vi "I2C Controller Module.vi"(11 "error in (no error)":errorcluster) -> (15 "error out":errorcluster)   [LabVIEW 2020, in "I2C Controller Lib.lvlib"]
uses:
  I2C Controller Lib.lvlib
  TypeDef/Transmission Data.ctl
  TypeDef/DVR Cluster.ctl
  Class/Transmission Mode/Parent/TX Speed.lvclass
  Class/Addressing Mode/Parent/Addressing Mode.lvclass
  Class/Devices/Parent/Devices.lvclass
  TypeDef/Path Cluster.ctl
  TypeDef/Queue Operation Mode.ctl
  TypeDef/User LV2 Mode Select.ctl
  <vilib>/Utility/config.llb/Read Key (String).vi
  Class/Transmission Mode/Child/Low Speed/SubVI/SubPanel.vi
  <vilib>/Utility/config.llb/NI_LVConfig.lvlib
  Class/Transmission Mode/Child/Low Speed/Low Speed.lvclass
panel:
  in  "Clear?":bool
  in  "Configure?":bool
  out "Warning":string caption="Warning:"
  in  "TX.Data":T1=[10, 188, 218, 14, 47, 69, 255, 107, 7, 92, 64] caption="Transmission Data" format="%.0x"
  out "RX.Data":u8[](array[numeric]) caption="Read Bytes" format="%.0x"
  out "Acknoledge?":bool caption="ACK / NACK"
  in  "Speed Mode":string(combo)="Select Device"
  in  "Transmit Data?":bool caption="Start Transmission"
  in  "Add Device?":bool caption="Add DEvice?"
  in  "Oper. Mode":string(combo)="Select Operation" caption="Operation Mode"
  in  "Address Mode":enum32{"7-bit", "10-Bit"}(radio) caption="Addressing Mode"
  in  "Log.Open?":bool
  in  "Target Address":u16 max=128 step=1 format="%.0x"
  in  "Device Type":string(combo)="Select Device Type"
  in  "Voltage":dbl=1.8 caption="Voltage (V)" min=1.8 max=5.0 step=1.0 format="%.2g"
  out "Digital Waveform Graph":digitaldata[](graph) caption="Graph"
  # "I2C Controller Module"
  # "Controller"
  # "Target"
  # "Transmission Parameters"
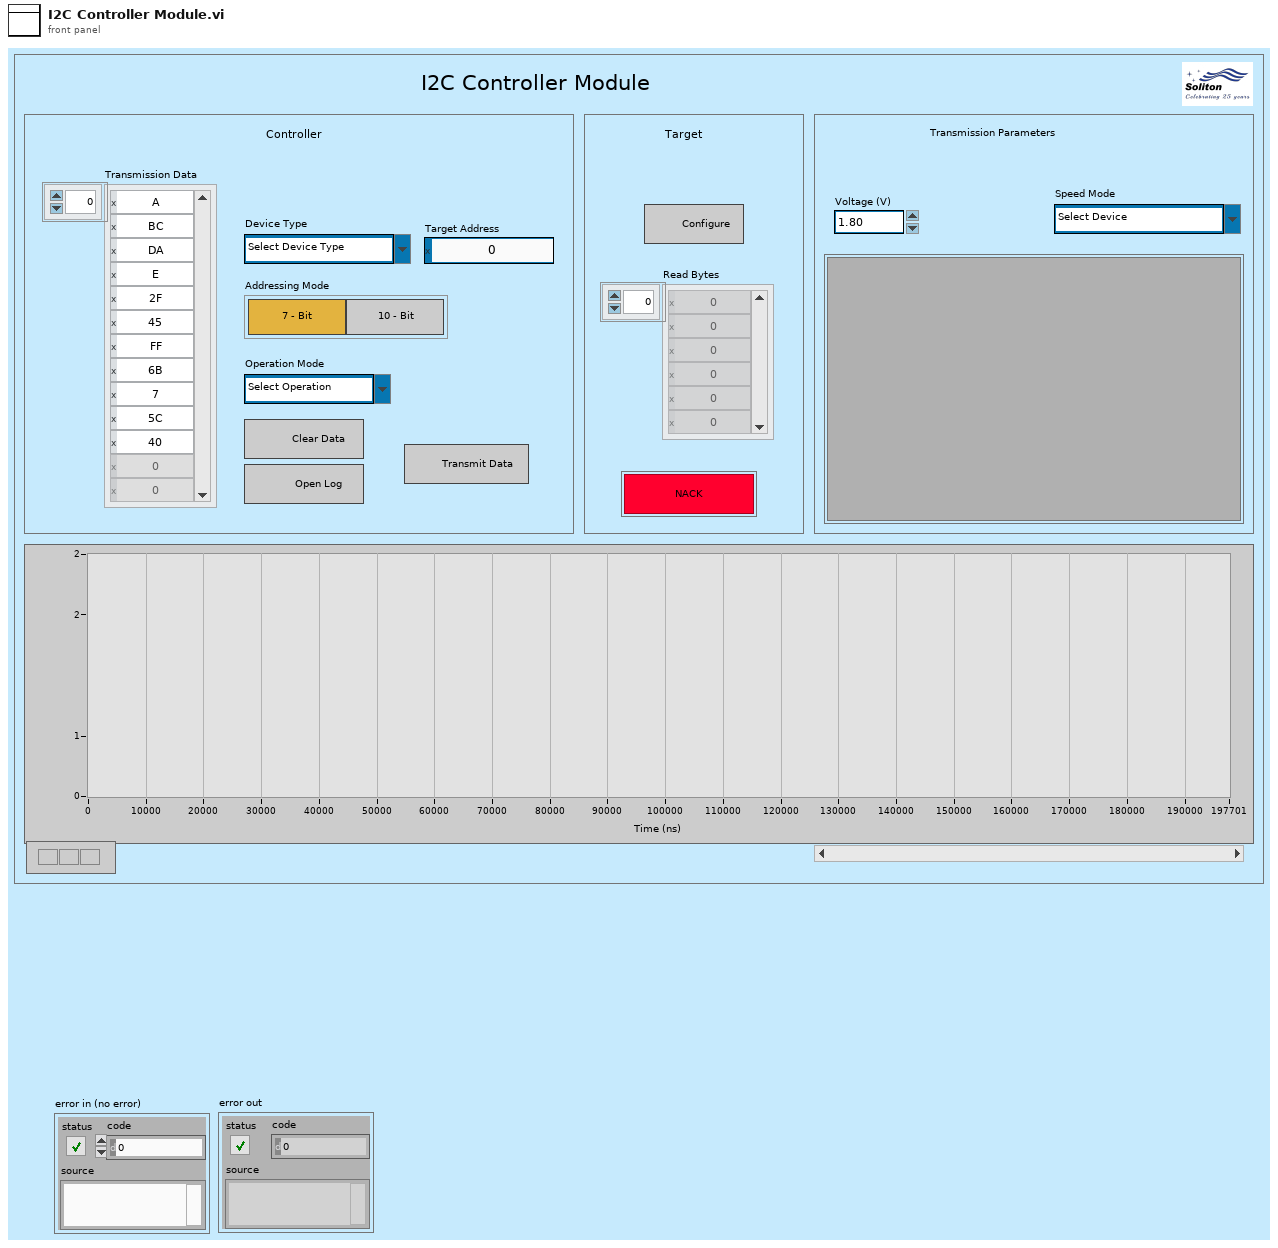
[diagram p1: front panel]
types:
  T1 = typedef "I2C Controller Lib.lvlib/Transmission Data.ctl" = u8[]
  T2 = typedef "I2C Controller Lib.lvlib/User LV2 Mode Select.ctl" = enum16{"Create", "Delete", "Stop"}
  T3 = typedef "I2C Controller Lib.lvlib/Queue Operation Mode.ctl" = enum16{"Create Q", "Enqueue", "Enqueue N", "Enstack", "Dequeue", "Flush Q", "Close Q"}
  T4 = typedef "I2C Controller Lib.lvlib/DVR Cluster.ctl" = cluster{"TX. Mode":refnum<data-value>, "Addr. Mode":refnum<data-value>, "Devices":refnum<data-value>}
  T5 = typedef "I2C Controller Lib.lvlib/Path Cluster.ctl" = cluster{"Config File":path, "TX.Mode":path, "Devices":path, "Addr. Mode":path}
  T6 = cluster{"Enable/Disable":string, "Warning":string, "Oper. Mode":string, "Speed Mode":string, "Address Mode":enum32{"7-bit", "10-Bit"}, "TX.Data":T1, "Device Type":string, "DVR":T4, "Path":T5, "Flags":cluster{"Device Type":bool, "Speed Mode":bool, "Target Address":bool, "Oper. Mode":bool}, "RX.Data":u8[], "Acknoledge?":bool, "Graph Wave":digitaldata[]}
  T7 = typedef "NI_LVConfig.lvlib/Config Data RefNum.ctl" = refnum<k1>
  T8 = enum8{"Enabled", "Disabled", "Disabled and Grayed Out"}
  T9 = cluster{"Device Type":bool, "Speed Mode":bool, "Target Address":bool, "Oper. Mode":bool}
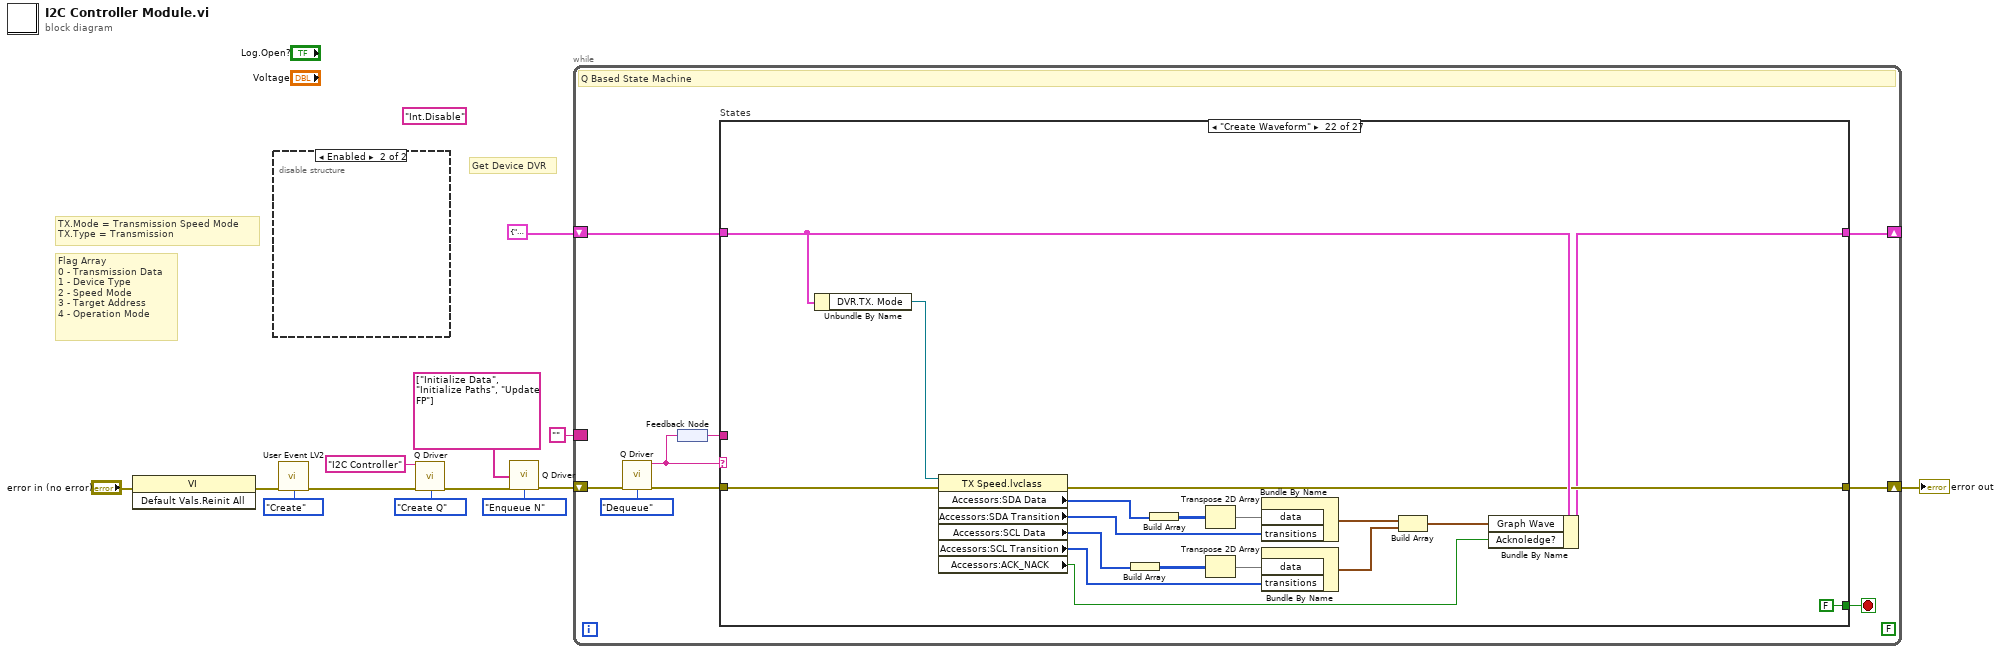
[diagram p0: block diagram]
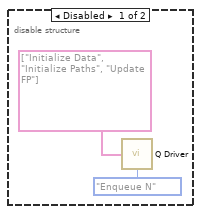
[diagram p2: hidden frame]
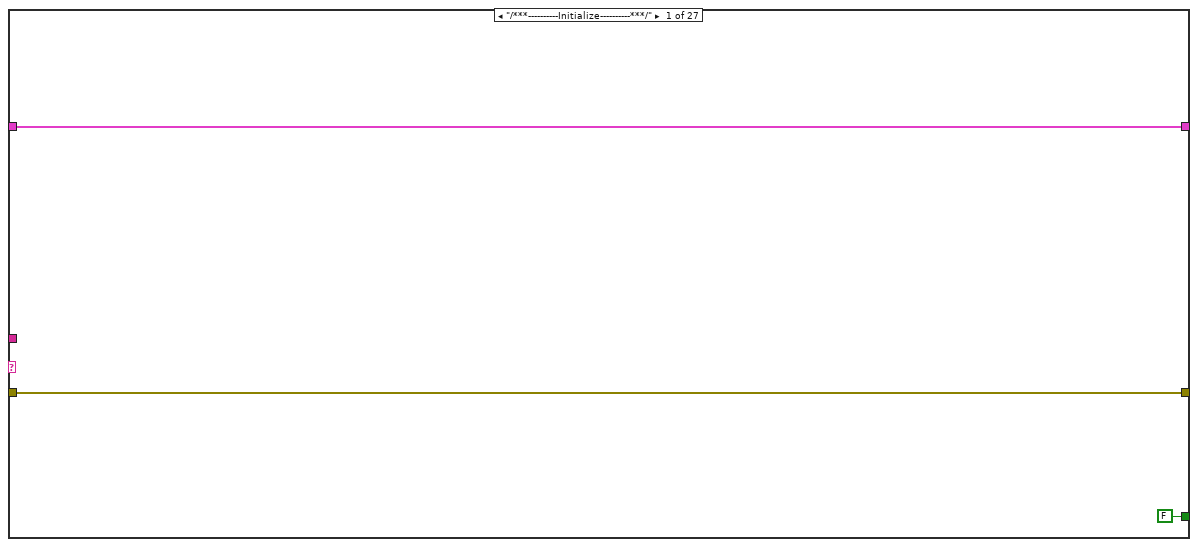
[diagram p3: hidden frame]
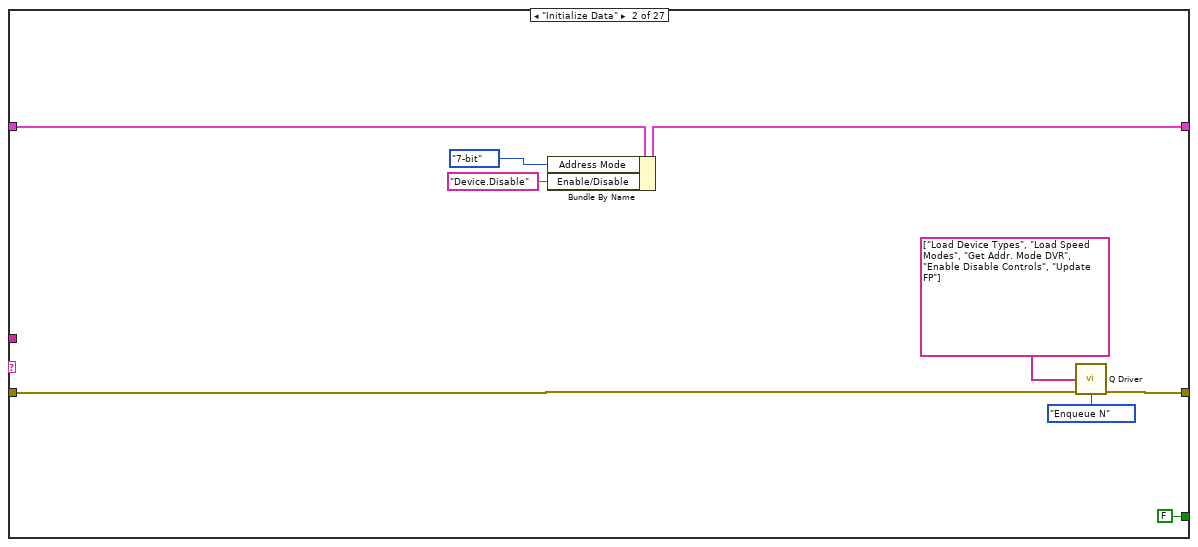
[diagram p4: hidden frame]
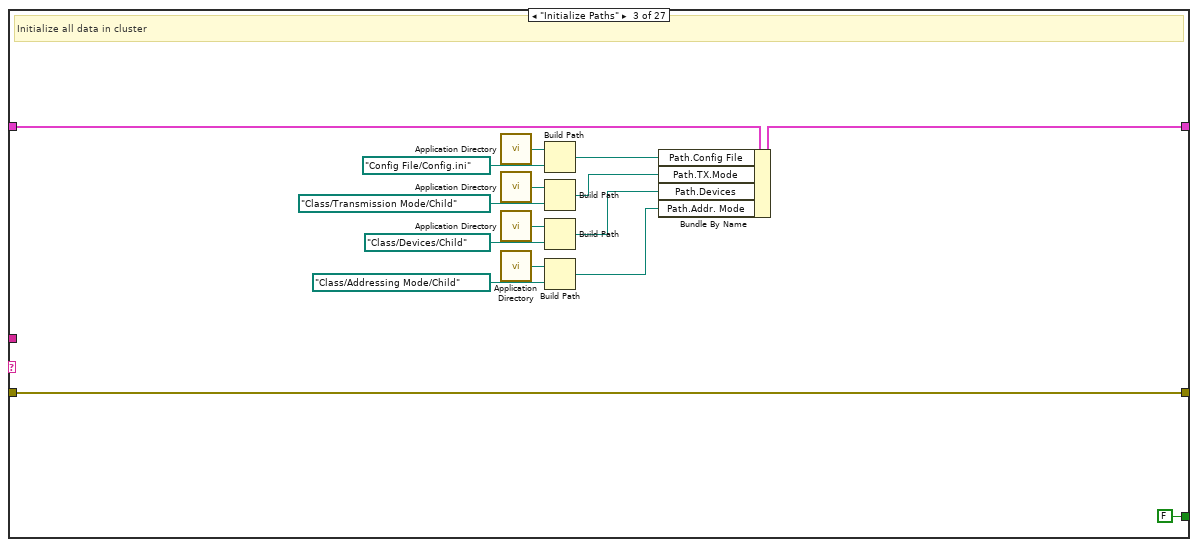
[diagram p5: hidden frame]
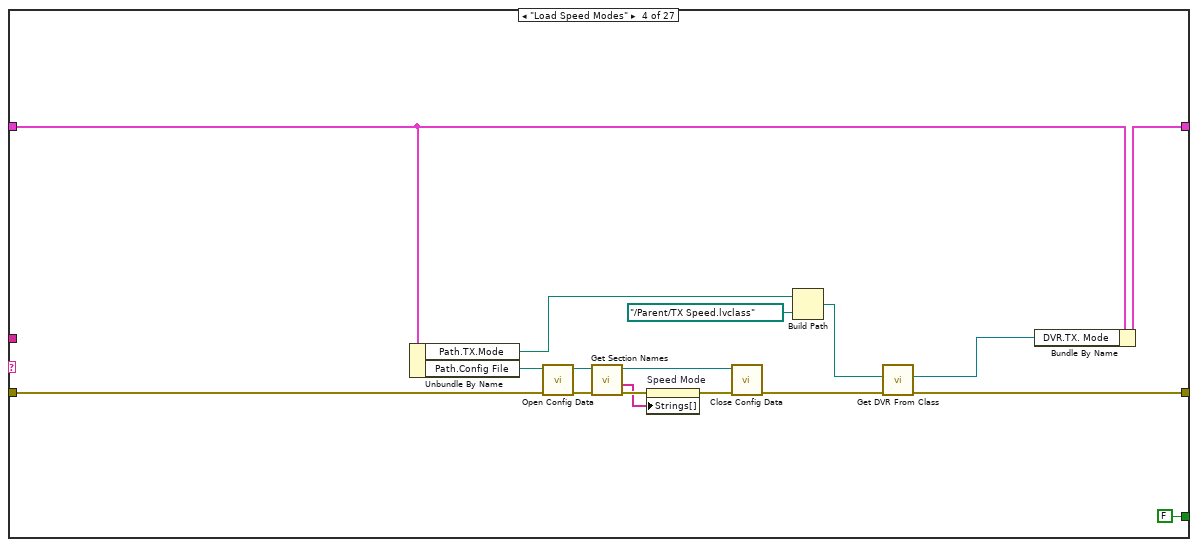
[diagram p6: hidden frame]
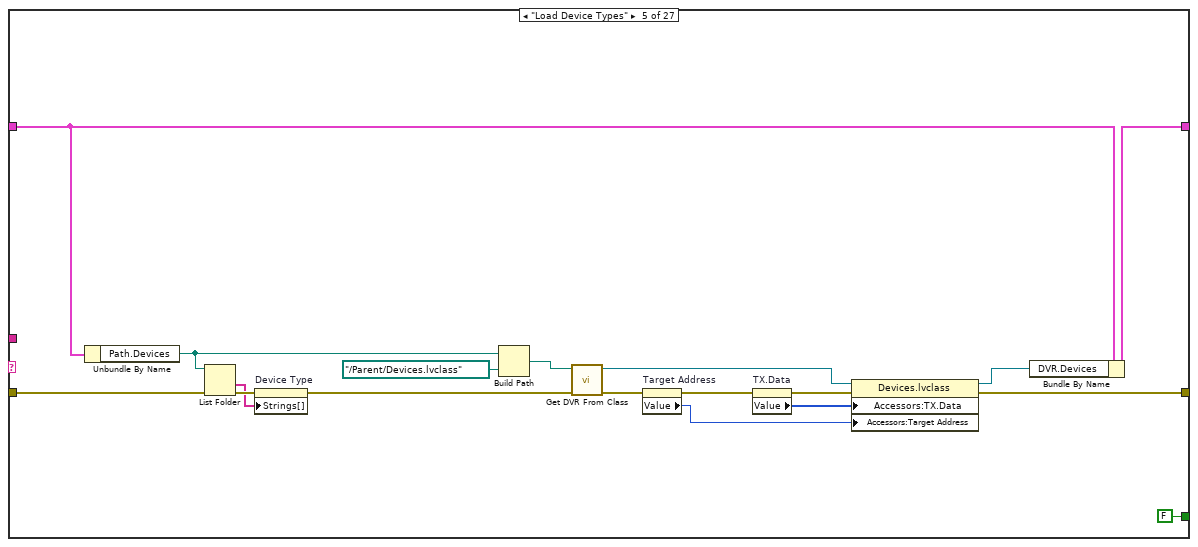
[diagram p7: hidden frame]
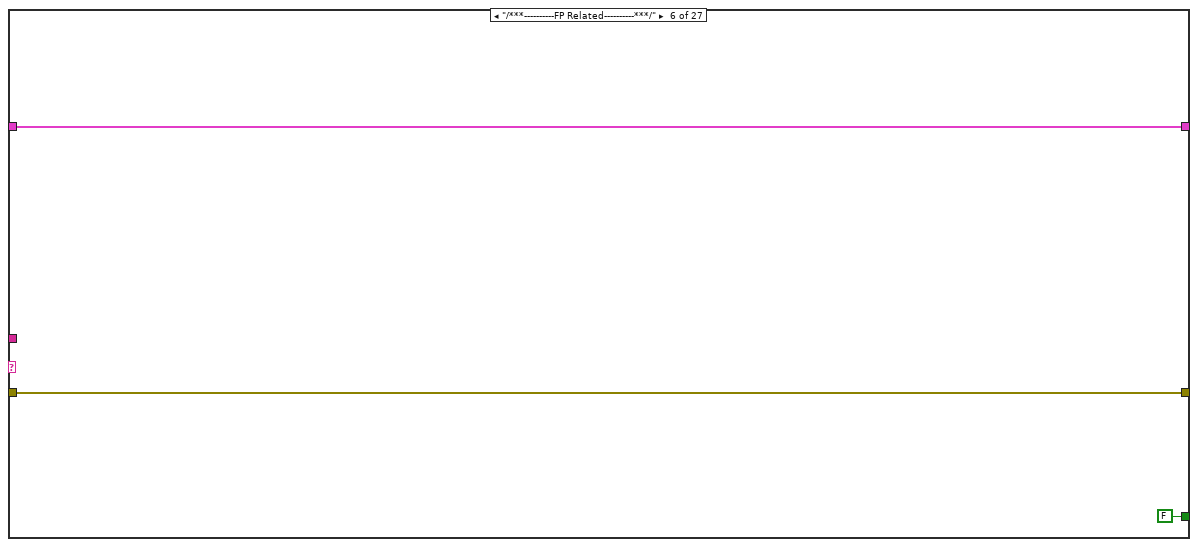
[diagram p8: hidden frame]
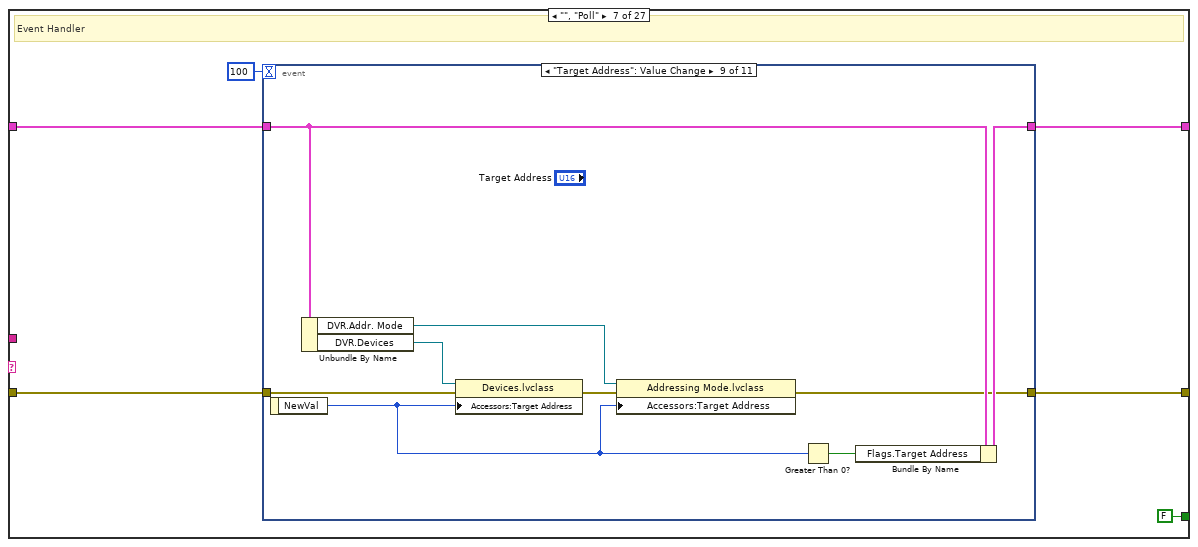
[diagram p9: hidden frame]
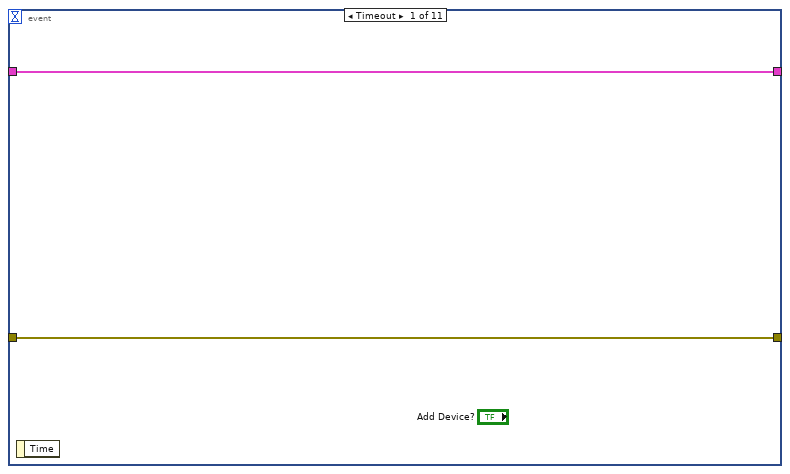
[diagram p10: hidden frame]
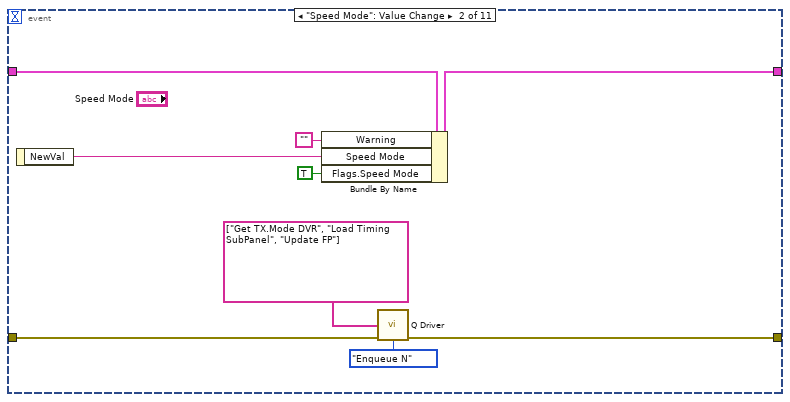
[diagram p11: hidden frame]
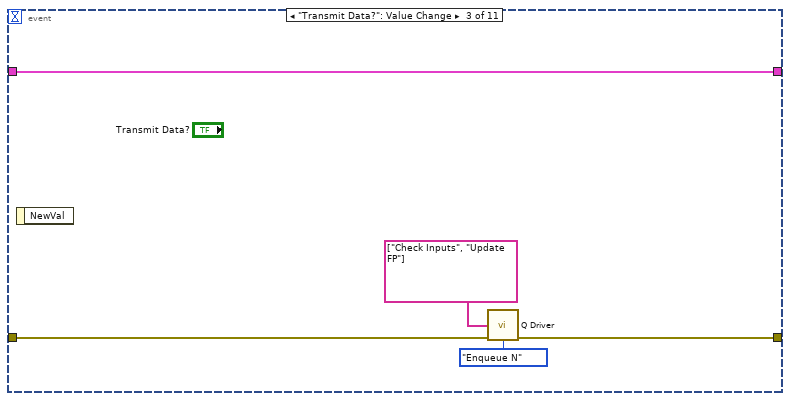
[diagram p12: hidden frame]
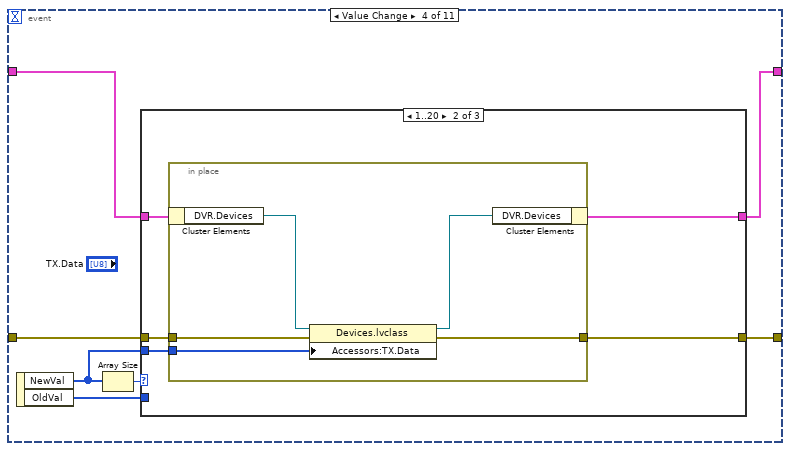
[diagram p13: hidden frame]
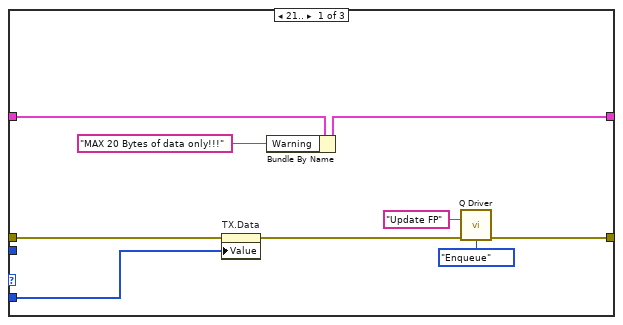
[diagram p14: hidden frame]
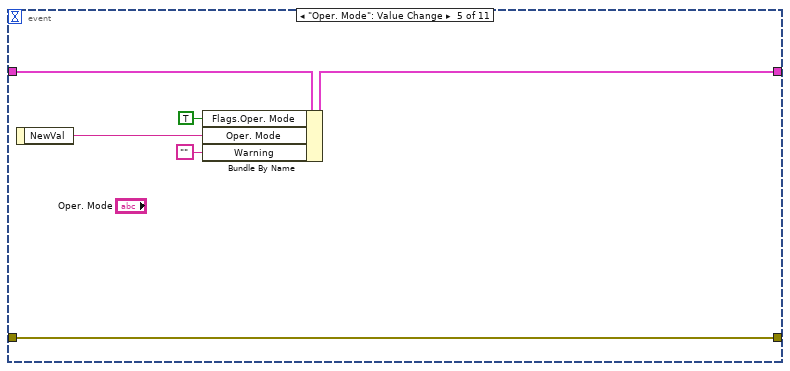
[diagram p16: hidden frame]
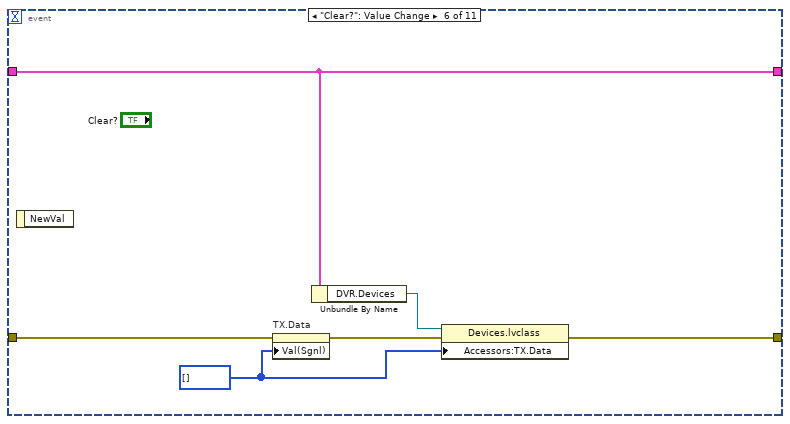
[diagram p17: hidden frame]
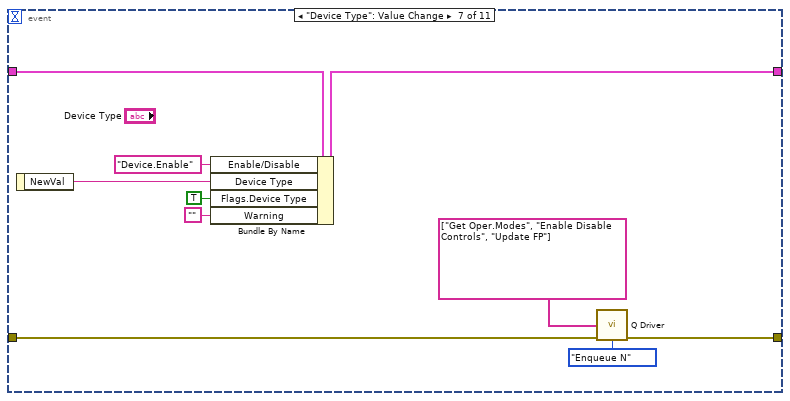
[diagram p18: hidden frame]
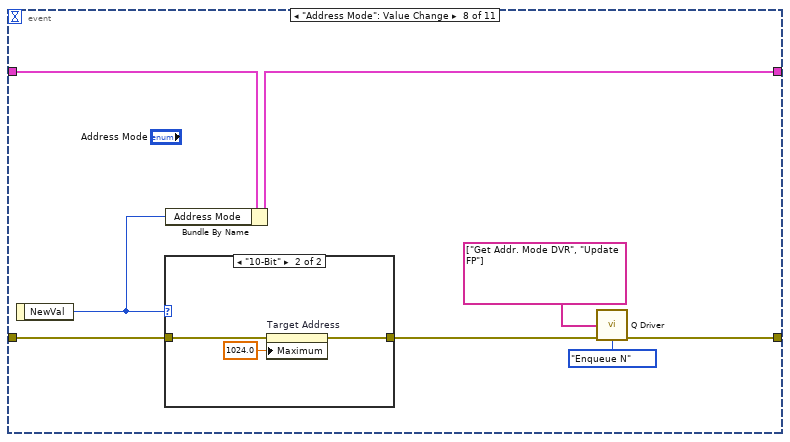
[diagram p19: hidden frame]
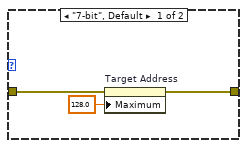
[diagram p20: hidden frame]
diagram:
  (unwired) "Int.Disable" ("Enable/Disable")
  # "Get Device DVR"
  # "Flag Array\n0 - Transmission Data\n1 - Device Type\n2 - Speed Mode\n3 - Target Address\n4 - Operation Mode"
  # "TX.Mode = Transmission Speed Mode\nTX.Type = Transmission"
  n1 = invoke class="VI" method="Default Vals.Reinit All"(error in="error in (no error)") -> (error out=w2:errorcluster)  [unwired: 2 in, 2 out]
  n2 = disable-structure shown="Enabled" {
    frame Disabled {
      n3 = call "Q Driver.vi"("States s[]"=string[] ["Initialize Data", "Initialize Paths", "Update FP"], "Q Operation"=Queue_Operation_Mode."Enqueue N") -> ()  [unwired: 12 in, 2 out]
    }
    frame Enabled {
    }
  }
  n4 = call "User Event LV2.vi"("error in (no error)"=w2, "LV2 Mode"=User_LV2_Mode_Select."Create") -> ("error out"=w1:errorcluster)  [unwired: 12 in, 1 out]
  n5 = call "Q Driver.vi"("Q Name"="I2C Controller", "error in (no error)"=w1, "Q Operation"=Queue_Operation_Mode."Create Q") -> ("error out"=w12:errorcluster)  [unwired: 11 in, 1 out]
  n6 = call "Q Driver.vi"("States s[]"=string[] ["Initialize Data", "Initialize Paths", "Update FP"], "error in (no error)"=w12, "Q Operation"=Queue_Operation_Mode."Enqueue N") -> ("error out"=w11:errorcluster)  [unwired: 11 in, 1 out]
  n7 = while {
    shift-right: [w21] -> _
    shift-left: T6 {"Enable/Disable"="", "Warning"="", "Oper. Mode"="", "Speed Mode"="", "Address Mode"=enum."7-bit", "TX.Data"=[], "Device Type"="", "DVR"={"TX. Mode"=refnum, "Addr. Mode"=refnum, "Devices"=refnum}, "Path"={"Config File"=path "", "TX.Mode"=path "", "Devices"=path "", "Addr. Mode"=path ""}, "Flags"={"Device Type"=FALSE, "Speed Mode"=FALSE, "Target Address"=FALSE, "Oper. Mode"=FALSE}, "RX.Data"=[], "Acknoledge?"=FALSE, "Graph Wave"=[]} -> [w20]
    shift-right: [w22] -> w8
    shift-left: w11 -> [w24]
    border: "" -> [_]
    stop <- w19 stop-if-true
    (unwired) FALSE
    (unwired) FALSE
    # "Q Based State Machine"
    n8 = call "Q Driver.vi"("error in (no error)"=w24, "Q Operation"=Queue_Operation_Mode."Dequeue") -> ("State Out"=w17:string, "error out"=w23:errorcluster)  [unwired: 12 in]
    n9 = feedback-in #1(w17) -> ()
    n10 = feedback #1() -> (w16:string)
    n11 = case "States" shown="\"Create Waveform\"" w17 {
      selector: w17 -> [_ _ _ _ _ _ _ _ _ _ _ _ _ _ _ _ _ _ _ _ _ _ _ _ w490 _ _]
      tunnel: w23 -> [w27 w31 w40 w68 w86 w90 w96 w213 w233 w236 w242 w272 w288 w308 w319 w325 w332 w351 w366 w394 w447 w465 w468 w471 w492 w513 w518]
      tunnel: [w27 w30 w40 w55 w75 w90 w95 w214 w233 w236 w244 w274 w285 w308 w318 w324 w331 w351 w358 w392 w436 w463 w468 w470 w491 w513 w516] -> w22
      tunnel: [w26 w35 w50 w54 w80 w89 w93 w212 w231 w235 w243 w275 w290 w307 w320 w323 w330 w350 w361 w395 w434 w451 w467 w482 w503 w512 w520] -> w21
      tunnel: w20 -> [w26 w36 w51 w61 w85 w89 w92 w212 w231 w235 w250 w273 w287 w307 w320 w323 w330 w350 w361 w397 w444 w464 w467 w482 w503 w512 w520]
      tunnel: [FALSE FALSE FALSE FALSE FALSE FALSE FALSE FALSE FALSE FALSE FALSE FALSE FALSE FALSE FALSE FALSE FALSE FALSE FALSE FALSE FALSE FALSE FALSE FALSE FALSE FALSE TRUE] -> w19
      tunnel: w16 -> [_ _ _ _ _ _ _ _ _ _ _ _ _ _ _ _ _ _ _ _ _ _ _ w469 _ _ _]
      frame "/***----------Initialize----------***/" {
      }
      frame "Initialize Data" {
        n12 = Bundle By Name(cluster=w36, "Address Mode"=enum32{"7-bit", "10-Bit"}."7-bit", "Enable/Disable"="Device.Disable") -> (w35:T6)
        n13 = call "Q Driver.vi"("States s[]"=string[] ["Load Device Types", "Load Speed Modes", "Get Addr. Mode DVR", "Enable Disable Controls", "Update FP"], "error in (no error)"=w31, "Q Operation"=Queue_Operation_Mode."Enqueue N") -> ("error out"=w30:errorcluster)  [unwired: 11 in, 1 out]
      }
      frame "Initialize Paths" {
        # "Initialize all data in cluster"
        n14 = call <vilib>:"Application Directory.vi"() -> ("Application Directory"=w49:path)
        n15 = call <vilib>:"Application Directory.vi"() -> ("Application Directory"=w45:path)
        n16 = call <vilib>:"Application Directory.vi"() -> ("Application Directory"=w43:path)
        n17 = call <vilib>:"Application Directory.vi"() -> ("Application Directory"=w39:path)
        n18 = Build Path(base path=w49, name or relative path=path "Config File/Config.ini" ("Config.ini")) -> (appended path=w47:path)
        n19 = Build Path(base path=w45, name or relative path=path "Class/Transmission Mode/Child" ("Config.ini")) -> (appended path=w44:path)
        n20 = Build Path(base path=w43, name or relative path=path "Class/Devices/Child" ("Config.ini")) -> (appended path=w41:path)
        n21 = Build Path(base path=w39, name or relative path=path "Class/Addressing Mode/Child" ("Config.ini")) -> (appended path=w37:path)
        n22 = Bundle By Name(cluster=w51, "Path.Config File"=w47, "Path.TX.Mode"=w44, "Path.Devices"=w41, "Path.Addr. Mode"=w37) -> (w50:T6)
      }
      frame "Load Speed Modes" {
        n23 = Unbundle By Name(w61) -> ("Path.TX.Mode"=w59:path, "Path.Config File"=w60:path)
        n24 = call <vilib>:"Open Config Data.vi"("error in (no error)"=w68, "configuration file path"=w60) -> ("error out"=w67:errorcluster, "refnum"=w66:T7)  [unwired: 7 in, 1 out]
        n25 = call <vilib>:"Get Section Names.vi"("error in (no error)"=w67, "refnum"=w66) -> ("error out"=w65:errorcluster, "section names"=w64:string[], "refnum out"=w62:T7)  [unwired: 7 in]
        n26 = property on="Speed Mode" class="CmbBox"(error in=w65, "Strings[]"=w64) -> (error out=w63:errorcluster)  [unwired: 1 in, 1 out]
        n27 = call <vilib>:"Close Config Data.vi"("error in (no error)"=w63, "refnum"=w62) -> ("error out"=w56:errorcluster)  [unwired: 8 in, 1 out]
        n28 = Build Path(base path=w59, name or relative path=path "../Parent/TX Speed.lvclass") -> (appended path=w57:path)
        n29 = call "Get DVR From Class.vi"("error in (no error)"=w56, "Path In"=w57) -> ("error out"=w55:errorcluster, "Class DVR"=w53:refnum<data-value>)  [unwired: 7 in, 1 out]
        n30 = Bundle By Name(cluster=w61, "DVR.TX. Mode"=w53) -> (w54:T6)
      }
      frame "Load Device Types" {
        n31 = Unbundle By Name(w85) -> ("Path.Devices"=w79:path)
        n32 = List Folder(path=w79, error in=w86) -> (folder names=w83:string[], error out=w84:errorcluster)  [unwired: 2 in, 2 out]
        n33 = property on="Device Type" class="CmbBox"(error in=w84, "Strings[]"=w83) -> (error out=w82:errorcluster)  [unwired: 1 in, 1 out]
        n34 = Build Path(base path=w79, name or relative path=path "../Parent/Devices.lvclass") -> (appended path=w78:path)
        n35 = call "Get DVR From Class.vi"("error in (no error)"=w82, "Path In"=w78) -> ("error out"=w81:errorcluster, "Devices DVR"=w74:refnum<data-value>)  [unwired: 8 in]
        n36 = property on="Target Address" class="DigNum (strict)"(error in=w81) -> (error out=w71:errorcluster, "Value"=w70:u16)  [unwired: 1 in, 1 out]
        n37 = property on="TX.Data" class="Arr (strict)"(error in=w71) -> (error out=w76:errorcluster, "Value"=w73:T1)  [unwired: 1 in, 1 out]
        n38 = property class="Devices.lvclass"(reference=w74, error in=w76, "Accessors:TX.Data"=w73, "Accessors:Target Address"=w70) -> (reference out=w72:refnum<data-value>, error out=w75:errorcluster)
        n39 = Bundle By Name(cluster=w85, "DVR.Devices"=w72) -> (w80:T6)
      }
      frame "/***----------FP Related----------***/" {
      }
      frame "", "Poll" {
        # "Event Handler"
        n40 = event shown="[8] \"Target Address\": Value Change" {
          selector: _ -> [_ _ _ _ _ _ _ _ _ _ _]
          dyn-events: _ -> [_ _ _ _ _ _ _ _ _ _ _]
          timeout: 100 -> [_ _ _ _ _ _ _ _ _ _ _]
          tunnel: w96 -> [w98 w103 w109 w119 w141 w152 w159 w169 w183 w192 w209]
          tunnel: [w98 w102 w108 w118 w141 w149 w158 w166 w177 w191 w208] -> w95
          tunnel: [w97 w106 w112 w113 w145 w150 w154 w164 w185 w189 w207] -> w93
          tunnel: w92 -> [w97 w107 w112 w117 w146 w150 w162 w170 w181 w188 w207]
          event Timeout {
            n41 = event-data() -> ()  [unwired: 1 in, 1 out]
          }
          event "Speed Mode": Value Change {
            n42 = event-data() -> ("NewVal"=w105:string)  [unwired: 1 in]
            n43 = Bundle By Name(cluster=w107, "Warning"="", "Speed Mode"=w105, "Flags.Speed Mode"=TRUE) -> (w106:T6)
            n44 = call "Q Driver.vi"("States s[]"=string[] ["Get TX.Mode DVR", "Load Timing SubPanel", "Update FP"], "error in (no error)"=w103, "Q Operation"=Queue_Operation_Mode."Enqueue N") -> ("error out"=w102:errorcluster)  [unwired: 11 in, 1 out]
          }
          event "Transmit Data?": Value Change {
            n45 = event-data() -> ()  [unwired: 1 in, 1 out]
            n46 = call "Q Driver.vi"("States s[]"=string[] ["Check Inputs", "Update FP"], "error in (no error)"=w109, "Q Operation"=Queue_Operation_Mode."Enqueue N") -> ("error out"=w108:errorcluster)  [unwired: 11 in, 1 out]
          }
          event Value Change {
            n47 = event-data() -> ("NewVal"=w116:T1, "OldVal"=w114:T1)  [unwired: 1 in]
            n48 = Array Size(array=w116) -> (size(s)=w115:i32)
            n49 = case shown="1..20" w115 {
              tunnel: w119 -> [w127 w133 w139]
              tunnel: [w125 w129 w140] -> w113
              tunnel: [w121 w132 w139] -> w118
              tunnel: w117 -> [w128 w130 w140]
              tunnel: w116 -> [_ w131 _]
              tunnel: w114 -> [w126 _ _]
              frame 21.. {
                n50 = property on="TX.Data" class="Arr (strict)"(error in=w127, "Value"=w126) -> (error out=w122:errorcluster)  [unwired: 1 in, 1 out]
                n51 = Bundle By Name(cluster=w128, "Warning"="MAX 20 Bytes of data only!!!") -> (w125:T6)
                n52 = call "Q Driver.vi"("State In"="Update FP" ("element"), "error in (no error)"=w122, "Q Operation"=Queue_Operation_Mode."Enqueue") -> ("error out"=w121:errorcluster)  [unwired: 11 in, 1 out]
              }
              frame 1..20 {
                n53 = in-place {
                  in-place-border: w133 -> [w138]
                  in-place-border: [w137] -> w132
                  in-place-border: w131 -> [w136]
                  n54 = in-place-cluster #2(w130) -> ("DVR.Devices"=w135:refnum<data-value>)
                  n55 = property class="Devices.lvclass"(reference=w135, error in=w138, "Accessors:TX.Data"=w136) -> (reference out=w134:refnum<data-value>, error out=w137:errorcluster)
                  n56 = in-place-cluster #2("DVR.Devices"=w134) -> (w129:T6)
                }
              }
              frame 0, Default {
              }
            }
          }
          event "Oper. Mode": Value Change {
            n57 = event-data() -> ("NewVal"=w143:string)  [unwired: 1 in]
            n58 = Bundle By Name(cluster=w146, "Flags.Oper. Mode"=TRUE, "Oper. Mode"=w143, "Warning"="") -> (w145:T6)
          }
          event "Clear?": Value Change {
            w147 = T1 [] ("TX.Data")
            n59 = event-data() -> ()  [unwired: 1 in, 1 out]
            n60 = property on="TX.Data" class="Arr (strict)"(error in=w152, "Val(Sgnl)"=w147) -> (error out=w151:errorcluster)  [unwired: 1 in, 1 out]
            n61 = Unbundle By Name(w150) -> ("DVR.Devices"=w148:refnum<data-value>)
            n62 = property class="Devices.lvclass"(reference=w148, error in=w151, "Accessors:TX.Data"=w147) -> (error out=w149:errorcluster)  [unwired: 1 out]
          }
          event "Device Type": Value Change {
            n63 = event-data() -> ("NewVal"=w161:string)  [unwired: 1 in]
            n64 = Bundle By Name(cluster=w162, "Enable/Disable"="Device.Enable", "Device Type"=w161, "Flags.Device Type"=TRUE, "Warning"="") -> (w154:T6)
            n65 = call "Q Driver.vi"("States s[]"=string[] ["Get Oper.Modes", "Enable Disable Controls", "Update FP"], "error in (no error)"=w159, "Q Operation"=Queue_Operation_Mode."Enqueue N") -> ("error out"=w158:errorcluster)  [unwired: 11 in, 1 out]
          }
          event "Address Mode": Value Change {
            n66 = event-data() -> ("NewVal"=w163:enum32{"7-bit", "10-Bit"})  [unwired: 1 in]
            n67 = case shown="\"10-Bit\"" w163 {
              tunnel: [w171 w175] -> w167
              tunnel: w169 -> [w172 w176]
              frame "7-bit", Default {
                n68 = property on="Target Address" class="DigNum (strict)"(error in=w172, "Maximum"=128.0 ("Data Entry Limits:Maximum")) -> (error out=w171:errorcluster)  [unwired: 1 in, 1 out]
              }
              frame "10-Bit" {
                n69 = property on="Target Address" class="DigNum (strict)"(error in=w176, "Maximum"=1024.0 ("Data Entry Limits:Maximum")) -> (error out=w175:errorcluster)  [unwired: 1 in, 1 out]
              }
            }
            n70 = Bundle By Name(cluster=w170, "Address Mode"=w163) -> (w164:T6)
            n71 = call "Q Driver.vi"("States s[]"=string[] ["Get Addr. Mode DVR", "Update FP"], "error in (no error)"=w167, "Q Operation"=Queue_Operation_Mode."Enqueue N") -> ("error out"=w166:errorcluster)  [unwired: 11 in, 1 out]
          }
          event "Target Address": Value Change {
            n72 = event-data() -> ("NewVal"=w178:u16)  [unwired: 1 in]
            n73 = Unbundle By Name(w181) -> ("DVR.Addr. Mode"=w179:refnum<data-value>, "DVR.Devices"=w180:refnum<data-value>)
            n74 = property class="Devices.lvclass"(reference=w180, error in=w183, "Accessors:Target Address"=w178) -> (error out=w182:errorcluster)  [unwired: 1 out]
            n75 = property class="Addressing Mode.lvclass"(reference=w179, error in=w182, "Accessors:Target Address"=w178) -> (error out=w177:errorcluster)  [unwired: 1 out]
            n76 = Greater Than 0?(x=w178) -> (x > 0?=w184:bool)
            n77 = Bundle By Name(cluster=w181, "Flags.Target Address"=w184) -> (w185:T6)
          }
          event "Configure?": Value Change {
            n78 = event-data() -> ()  [unwired: 1 in, 1 out]
            n79 = Unbundle By Name(w188) -> ("Flags.Device Type"=w190:bool, "Flags.Oper. Mode"=w186:bool)
            n80 = And(x=w190, y=w186) -> (x .and. y?=w187:bool)
            n81 = case shown="True" w187 {
              tunnel: w192 -> [w195 w203]
              tunnel: [w194 w202] -> w191
              tunnel: [w198 w200] -> w189
              tunnel: w188 -> [w199 w200]
              frame False {
                n82 = call "Q Driver.vi"("State In"="Update FP" ("element"), "error in (no error)"=w195, "Q Operation"=Queue_Operation_Mode."Enqueue") -> ("error out"=w194:errorcluster)  [unwired: 11 in, 1 out]
                n83 = Bundle By Name(cluster=w199, "Warning"="Select Device Type and Operation Mode") -> (w198:T6)
              }
              frame True {
                n84 = call "Q Driver.vi"("States s[]"=string[] ["Get Device DVR", "Config RX data", "Update FP"], "error in (no error)"=w203, "Q Operation"=Queue_Operation_Mode."Enqueue N") -> ("error out"=w202:errorcluster)  [unwired: 11 in, 1 out]
              }
            }
          }
          event Panel Close? {
            n85 = event-data() -> ()  [unwired: 1 in, 1 out]
            n86 = call "Q Driver.vi"("State In"="Exit" ("Q Name"), "error in (no error)"=w209, "Q Operation"=Queue_Operation_Mode."Enqueue") -> ("error out"=w208:errorcluster)  [unwired: 11 in, 1 out]
            n87 = event-data("Discard?"=TRUE) -> ()  [unwired: 1 in, 1 out]
          }
        }
      }
      frame "Enable Disable Controls" {
        # "Enable Disable required controls"
        n88 = Unbundle By Name(w212) -> ("Enable/Disable"=w211:string)
        n89 = case shown="\"Device.Disable\"" w211 {
          tunnel: [w216 w218 w222] -> w214
          tunnel: w213 -> [w216 w221 w225]
          frame Default {
          }
          frame "Device.Enable" {
            w217 = T8."Enabled" ("Disabled")
            n90 = property on="Target Address" class="DigNum (strict)"(error in=w221, "DisabledEnum"=w217) -> (error out=w220:errorcluster)  [unwired: 1 in, 1 out]
            n91 = property on="Address Mode" class="RadioBtnsControl (strict)"(error in=w220, "DisabledEnum"=w217) -> (error out=w219:errorcluster)  [unwired: 1 in, 1 out]
            n92 = property on="Oper. Mode" class="CmbBox"(error in=w219, "DisabledEnum"=w217) -> (error out=w218:errorcluster)  [unwired: 1 in, 1 out]
          }
          frame "Device.Disable" {
            w226 = T8."Disabled and Grayed Out" ("Disabled")
            n93 = property on="Target Address" class="DigNum (strict)"(error in=w225, "DisabledEnum"=w226) -> (error out=w224:errorcluster)  [unwired: 1 in, 1 out]
            n94 = property on="Address Mode" class="RadioBtnsControl (strict)"(error in=w224, "DisabledEnum"=w226) -> (error out=w223:errorcluster)  [unwired: 1 in, 1 out]
            n95 = property on="Oper. Mode" class="CmbBox"(error in=w223, "DisabledEnum"=w226) -> (error out=w222:errorcluster)  [unwired: 1 in, 1 out]
          }
        }
      }
      frame "Update FP" {
        # "Update Front Panel Controls and Indicators"
        n96 = Unbundle By Name(w231) -> ("Warning"=→"Warning":string, "RX.Data"=→"RX.Data":u8[], "Acknoledge?"=→"Acknoledge?":bool, "Graph Wave"=→"Digital Waveform Graph":digitaldata[])
      }
      frame "/***----------DVR Functions----------***/" {
      }
      frame "Get Addr. Mode DVR" {
        n97 = Unbundle By Name(w250) -> ("Path.Addr. Mode"=w248:path, "Address Mode"=w237:enum32{"7-bit", "10-Bit"}, "DVR.Addr. Mode"=w240:refnum<data-value>)
        n98 = call "Close DVR Referance.vi"("error in (no error)"=w242, "Addr. Mode DVR"=w240) -> ("error out"=w241:errorcluster)  [unwired: 9 in]
        n99 = Path To String(path=w248) -> (string=w249:string)
        n100 = Format Into String(format string="\\\\%s\\\\%s.lvclass", initial string=w249, error in=w241, w237, w237) -> (resulting string=w246:string, error out=w245:errorcluster)
        n101 = String To Path(string=w246) -> (path=w238:path)
        n102 = call "Get DVR From Class.vi"("error in (no error)"=w245, "Path In"=w238) -> ("error out"=w244:errorcluster, "Addr. Mode DVR"=w239:refnum<data-value>)  [unwired: 8 in]
        n103 = Bundle By Name(cluster=w250, "DVR.Addr. Mode"=w239) -> (w243:T6)
      }
      frame "Get Device DVR" {
        n104 = Unbundle By Name(w273) -> ("Path.Devices"=w265:path, "Device Type"=w257:string, "Oper. Mode"=w256:string, "DVR.Devices"=w263:refnum<data-value>)
        n105 = property class="Devices.lvclass"(reference=w263, error in=w272) -> (reference out=w259:refnum<data-value>, error out=w261:errorcluster, "Accessors:TX.Data"=w262:T1, "Accessors:RX.Data"=w255:u8[], "Accessors:Target Address"=w254:u16, "Accessors:TX. Mode"=w253:refnum<data-value>, "Accessors:Addr. Mode"=w252:refnum<data-value>)
        n106 = call "Close DVR Referance.vi"("error in (no error)"=w261, "Devices DVR"=w259) -> ("error out"=w260:errorcluster)  [unwired: 9 in]
        n107 = Path To String(path=w265) -> (string=w271:string)
        n108 = Format Into String(format string="\\\\%s\\\\Child\\\\%s\\\\%s.lvclass", initial string=w271, error in=w260, w257, w256, w256) -> (resulting string=w268:string, error out=w269:errorcluster)
        n109 = String To Path(string=w268) -> (path=w266:path)
        n110 = call "Get DVR From Class.vi"("error in (no error)"=w269, "Path In"=w266) -> ("error out"=w267:errorcluster, "Devices DVR"=w264:refnum<data-value>)  [unwired: 8 in]
        n111 = property class="Devices.lvclass"(reference=w264, error in=w267, "Accessors:TX.Data"=w262, "Accessors:RX.Data"=w255, "Accessors:Target Address"=w254, "Accessors:TX. Mode"=w253, "Accessors:Addr. Mode"=w252) -> (reference out=w258:refnum<data-value>, error out=w274:errorcluster)
        n112 = Bundle By Name(cluster=w273, "DVR.Devices"=w258) -> (w275:T6)
      }
      frame "Get TX.Mode DVR" {
        n113 = Unbundle By Name(w287) -> ("DVR.TX. Mode"=w280:refnum<data-value>)
        n114 = property class="TX Speed.lvclass"(reference=w280, error in=w288) -> (reference out=w277:refnum<data-value>, error out=w279:errorcluster, "Accessors:Target Address"=w283:u16, "Accessors:ACK_NACK"=w281:bool)
        n115 = call "Close DVR Referance.vi"("error in (no error)"=w279, "DVR IN"=w277) -> ("error out"=w278:errorcluster)  [unwired: 9 in]
        n116 = Unbundle By Name(w287) -> ("Path.TX.Mode"=w299:path, "Speed Mode"=w301:string, "Path.Config File"=w302:path)
        n117 = call <vilib>:"Open Config Data.vi"("error in (no error)"=w278, "configuration file path"=w302) -> ("error out"=w305:errorcluster, "refnum"=w303:T7)  [unwired: 7 in, 1 out]
        n118 = Path To String(path=w299) -> (string=w298:string)
        n119 = call-poly <vilib>:"Read Key.vi"("section"=w301, "error in (no error)"=w305, "key"="Class", "refnum"=w303) -> ("error out"=w304:errorcluster, "value"=w286:string, "refnum out"=w295:T7)  [unwired: 4 in, 1 out]
        n120 = Format Into String(format string="\\\\%s\\\\%s.lvclass", initial string=w298, error in=w304, w286, w286) -> (resulting string=w292:string, error out=w296:errorcluster)
        n121 = String To Path(string=w292) -> (path=w291:path)
        n122 = call <vilib>:"Close Config Data.vi"("error in (no error)"=w296, "refnum"=w295) -> ("error out"=w294:errorcluster)  [unwired: 8 in, 1 out]
        n123 = call "Get DVR From Class.vi"("error in (no error)"=w294, "Path In"=w291) -> ("error out"=w293:errorcluster, "Class DVR"=w284:refnum<data-value>)  [unwired: 7 in, 1 out]
        n124 = property class="TX Speed.lvclass"(reference=w284, error in=w293, "Accessors:Target Address"=w283, "Accessors:ACK_NACK"=w281) -> (reference out=w282:refnum<data-value>, error out=w285:errorcluster)
        n125 = Bundle By Name(cluster=w287, "DVR.TX. Mode"=w282) -> (w290:T6)
      }
      frame "/***----------Device Type Functions----------***/" {
      }
      frame "Get Oper.Modes" {
        n126 = Unbundle By Name(w320) -> ("Path.Devices"=w314:path, "Device Type"=w312:string)
        n127 = Path To String(path=w314) -> (string=w313:string)
        n128 = Format Into String(format string="\\\\%s\\\\Child", initial string=w313, error in=w319, w312) -> (resulting string=w310:string, error out=w315:errorcluster)
        n129 = String To Path(string=w310) -> (path=w309:path)
        n130 = List Folder(path=w309, error in=w315) -> (folder names=w316:string[], error out=w317:errorcluster)  [unwired: 2 in, 2 out]
        n131 = property on="Oper. Mode" class="CmbBox"(error in=w317, "Strings[]"=w316) -> (error out=w318:errorcluster)  [unwired: 1 in, 1 out]
      }
      frame "Config RX data" {
        n132 = Unbundle By Name(w323) -> ("DVR.Devices"=w322:refnum<data-value>)
        n133 = call "SubVI Config API.vi"("error in (no error)"=w325, "Devices DVR In"=w322) -> ("error out"=w324:errorcluster)  [unwired: 8 in, 1 out]
      }
      frame "Check Address" {
        n134 = Unbundle By Name(w330) -> ("DVR.TX. Mode"=w328:refnum<data-value>, "DVR.Devices"=w327:refnum<data-value>)
        n135 = property class="Devices.lvclass"(reference=w327, error in=w332) -> (error out=w346:errorcluster, "Accessors:Target Address"=w339:u16)  [unwired: 1 out]
        n136 = call <vilib>:"Application Directory.vi"() -> ("Application Directory"=w348:path)
        n137 = Number To Hexadecimal String(2:w339) -> (0:w338:string)  [unwired: 1 in]
        n138 = Build Path(base path=w348, name or relative path=path "Config file/Allowed Targets.txt" ("Application Directory")) -> (appended path=w345:path)
        n139 = Open/Create/Replace File(file path (use dialog)=w345, error in=w346) -> (refnum out=w343:refnum<file>, error out=w344:errorcluster)  [unwired: 4 in, 1 out]
        n140 = Read from Text File(file (use dialog)=w343, error in=w344) -> (text=w342:string, error out=w334:errorcluster)  [unwired: 2 in, 2 out]
        n141 = Spreadsheet String To Array(delimiter (Tab)=",", format string="%s", spreadsheet string=w342, array type (2D Dbl)=string[] [] ("text")) -> (array=w340:string[])
        n142 = Search 1D Array(1D array=w340, element=w338) -> (index of element=w337:i32)  [unwired: 1 in]
        n143 = Greater Or Equal To 0?(x=w337) -> (x >= 0?=w333:bool)
        n144 = property class="TX Speed.lvclass"(reference=w328, error in=w334, "Accessors:ACK_NACK"=w333) -> (error out=w331:errorcluster)  [unwired: 1 out]
      }
      frame "/***----------Program Functionality----------***/" {
      }
      frame "Load Timing SubPanel" {
        n145 = call "User Event LV2.vi"("error in (no error)"=w366, "LV2 Mode"=User_LV2_Mode_Select."Stop") -> ("error out"=w359:errorcluster)  [unwired: 12 in, 1 out]
        n146 = Unbundle By Name(w361) -> ("Path.TX.Mode"=w375:path, "Speed Mode"=w377:string, "Path.Config File"=w378:path)
        n147 = call <vilib>:"Open Config Data.vi"("error in (no error)"=w359, "configuration file path"=w378) -> ("error out"=w381:errorcluster, "refnum"=w379:T7)  [unwired: 7 in, 1 out]
        n148 = Path To String(path=w375) -> (string=w374:string)
        n149 = call-poly <vilib>:"Read Key.vi"("section"=w377, "error in (no error)"=w381, "key"="Class", "refnum"=w379) -> ("error out"=w380:errorcluster, "value"=w372:string, "refnum out"=w367:T7)  [unwired: 4 in, 1 out]
        n150 = Unbundle By Name(w361) -> ("DVR.TX. Mode"=w360:refnum<data-value>, "Speed Mode"=w352:string)
        n151 = Format Into String(format string="\\\\%s\\\\SubVI\\\\SubPanel.vi", initial string=w374, error in=w380, w372) -> (resulting string=w370:string, error out=w369:errorcluster)
        n152 = String To Path(string=w370) -> (path=w363:path)
        n153 = vi-ref "Low Speed.lvclass:SubPanel.vi"() -> (w355:refnum<vi>)
        n154 = Open VI Reference(type specifier VI Refnum (for type only)=w355, vi path=w363, options=256, error in (no error)=w369) -> (vi reference=w354:refnum<vi>, error out=w364:errorcluster)  [unwired: 2 in]
        n155 = call-by-ref "Start Asynchronous Call"(reference=w354, error in=w364, "DVR In"=w360, "Speed Mode"=w352) -> (error out=w357:errorcluster)  [unwired: 12 in, 3 out]
        n156 = Open VI Reference(vi path=w363, error in (no error)=w357) -> (vi reference=w353:refnum<vi>, error out=w362:errorcluster)  [unwired: 4 in]
        n157 = invoke on="Timing Panel" class="SubPnl" method="Insert VI"(error in=w362, "VI Ref"=w353) -> (error out=w371:errorcluster)  [unwired: 2 in, 3 out]
        n158 = Close Reference(reference=w353, error in (no error)=w371) -> (error out=w368:errorcluster)
        n159 = call <vilib>:"Close Config Data.vi"("error in (no error)"=w368, "refnum"=w367) -> ("error out"=w358:errorcluster)  [unwired: 8 in, 1 out]
      }
      frame "Check Inputs" {
        n160 = Unbundle By Name(w397) -> ("Flags"=w396:T9, "DVR.Devices"=w388:refnum<data-value>)
        n161 = property class="Devices.lvclass"(reference=w388, error in=w394) -> (error out=w389:errorcluster, "Accessors:TX.Data"=w387:T1, "Accessors:RX.Data"=w386:u8[])  [unwired: 1 out]
        n162 = Cluster To Array(cluster=w396) -> (array=w391:bool[])
        n163 = And Array Elements(Boolean array=w391) -> (logical AND=w393:bool)
        n164 = Empty Array?(array=w387) -> (empty?=w384:bool)
        n165 = Empty Array?(array=w386) -> (empty?=w385:bool)
        n166 = And(x=w384, y=w385) -> (x .and. y?=w383:bool)
        n167 = case shown="True" w393 {
          tunnel: [w401 w424] -> w392
          tunnel: w389 -> [w401 w425]
          tunnel: w391 -> [w400 _]
          tunnel: [w399 w423] -> w390
          tunnel: w383 -> [_ w422]
          frame False {
            n168 = for {
              tunnel: w400 -> [w404] mode=indexing
              tunnel: [w403] -> w399
              i -> [w405]
              stop <- w402 stop-if-true
              n169 = Not(x=w404) -> (.not. x?=w402:bool)
              n170 = case shown="2" w405 {
                tunnel: [w408 w412 w416 w420] -> w403
                tunnel: w404 -> [w409 w413 w417 w421]
                frame 0, Default {
                  n171 = Select(t="", s=w409, f="Select Device Type") -> (s? t:f=w408:string)
                }
                frame 1 {
                  n172 = Select(t="", s=w413, f="Select Speed Mode") -> (s? t:f=w412:string)
                }
                frame 2 {
                  n173 = Select(t="", s=w417, f="Target Address Invalid") -> (s? t:f=w416:string)
                }
                frame 3 {
                  n174 = Select(t="", s=w421, f="Select Operation Mode") -> (s? t:f=w420:string)
                }
              }
            }
          }
          frame True {
            n175 = case shown="False" w422 {
              tunnel: w425 -> [w428 w431]
              tunnel: [w427 w431] -> w424
              tunnel: ["Transmission Started" "Both TX and RX Data is empty!!!"] -> w423
              frame False {
                # "All inputs present - Transmit data"
                n176 = call "Q Driver.vi"("States s[]"=string[] ["Get Device DVR", "Check Address", "Transmit Data", "Create Waveform", "Update FP"], "error in (no error)"=w428, "Q Operation"=Queue_Operation_Mode."Enqueue N") -> ("error out"=w427:errorcluster)  [unwired: 11 in, 1 out]
              }
              frame True {
                # "Both TX and RX Data is empty!!!"
              }
            }
          }
        }
        n177 = Bundle By Name(cluster=w397, "Warning"=w390) -> (w395:T6)
      }
      frame "Transmit Data" {
        n178 = Unbundle By Name(w444) -> ("DVR.Addr. Mode"=w443:refnum<data-value>, "DVR.TX. Mode"=w442:refnum<data-value>)
        n179 = Unbundle By Name(w444) -> ("DVR.Devices"=w441:refnum<data-value>)
        n180 = property class="Devices.lvclass"(reference=w441, error in=w447, "Accessors:Addr. Mode"=w443, "Accessors:TX. Mode"=w442) -> (reference out=w440:refnum<data-value>, error out=w438:errorcluster)
        n181 = call "Check Read_Write API.vi"("error in (no error)"=w438, "Devices DVR In"=w440) -> ("error out"=w437:errorcluster, "Devices DVR Out"=w439:refnum<data-value>)  [unwired: 8 in]
        n182 = call "Calculate I2C API.vi"("error in (no error)"=w437, "Devices DVR In"=w439) -> ("error out"=w445:errorcluster, "Devices DVR Out"=w435:refnum<data-value>)  [unwired: 8 in]
        n183 = property class="Devices.lvclass"(reference=w435, error in=w445) -> (error out=w436:errorcluster, "Accessors:RX.Data"=w433:u8[])  [unwired: 1 out]
        n184 = Bundle By Name(cluster=w444, "RX.Data"=w433) -> (w434:T6)
      }
      frame "Create Waveform" {
        n185 = Unbundle By Name(w464) -> ("DVR.TX. Mode"=w462:refnum<data-value>)
        n186 = property class="TX Speed.lvclass"(reference=w462, error in=w465) -> (error out=w463:errorcluster, "Accessors:SDA Data"=w454:u8[], "Accessors:SDA Transition"=w461:u32[], "Accessors:SCL Data"=w456:u8[], "Accessors:SCL Transition"=w455:u32[], "Accessors:ACK_NACK"=w448:bool)  [unwired: 1 out]
        n187 = Build Array(w456) -> (w457:u8[][])
        n188 = Build Array(w454) -> (w460:u8[][])
        n189 = Transpose 2D Array(2D array=w460) -> (transposed array=w459:u8[][])
        n190 = Transpose 2D Array(2D array=w457) -> (transposed array=w458:u8[][])
        n191 = Bundle By Name("data"=w459, "transitions"=w461) -> (w453:digitaldata)  [unwired: 1 in]
        n192 = Bundle By Name("data"=w458, "transitions"=w455) -> (w452:digitaldata)  [unwired: 1 in]
        n193 = Build Array(w453, w452) -> (w450:digitaldata[])
        n194 = Bundle By Name(cluster=w464, "Graph Wave"=w450, "Acknoledge?"=w448) -> (w451:T6)
      }
      frame "/***----------Error----------***/" {
      }
      frame "Error" {
        # "Handle Errors"
        n195 = Unbundle By Name(w471) -> ("code"=w478:i32, "source"=w477:string)
        n196 = call <vilib>:"Clear Errors.vi"("error in (no error)"=w471, "specific error code to clear (0: all)"=w478) -> ("error out"=w480:errorcluster)  [unwired: 4 in, 1 out]
        n197 = Format Into String(format string="PROGRAM ERROR\nState \"%s\".\nError Code: %d\nError Source: %s\n\nDo you wish to continue?", error in=w480, w469, w478, w477) -> (resulting string=w476:string, error out=w472:errorcluster)  [unwired: 1 in]
        n198 = Two Button Dialog(message=w476, 1:"Exit" ("F button name (\"Cancel\")"), 2:"Continue" ("T button name (\"OK\")")) -> (T button?=w473:bool)
        n199 = case "Continue?" shown="True" w473 {
          tunnel: w472 -> [w488 w489]
          tunnel: [w485 w489] -> w470
          frame False {
            # "Exit"
            n200 = call "Q Driver.vi"("error in (no error)"=w488, "Q Operation"=Queue_Operation_Mode."Flush Q") -> ("error out"=w486:errorcluster)  [unwired: 12 in, 1 out]
            n201 = call "Q Driver.vi"("State In"="Exit" ("States[]"), "error in (no error)"=w486, "Q Operation"=Queue_Operation_Mode."Enqueue") -> ("error out"=w485:errorcluster)  [unwired: 11 in, 1 out]
          }
          frame True {
            # "Continue"
          }
        }
      }
      frame "Developer Error", Default {
        # "Handle Errors"
        n202 = Unbundle By Name(w492) -> ("code"=w499:i32, "source"=w498:string)
        n203 = call <vilib>:"Clear Errors.vi"("error in (no error)"=w492, "specific error code to clear (0: all)"=w499) -> ("error out"=w501:errorcluster)  [unwired: 4 in, 1 out]
        n204 = Format Into String(format string="DEVELOPER ERROR\nState \"%s\" not found!!\nError Code: %d\nError Source: %s\n\nDo you wish to continue?", error in=w501, w490, w499, w498) -> (resulting string=w497:string, error out=w493:errorcluster)  [unwired: 1 in]
        n205 = Two Button Dialog(message=w497, 1:"Exit" ("F button name (\"Cancel\")"), 2:"Continue" ("T button name (\"OK\")")) -> (T button?=w494:bool)
        n206 = case "Continue?" shown="False" w494 {
          tunnel: w493 -> [w509 w510]
          tunnel: [w506 w510] -> w491
          frame False {
            # "Exit"
            n207 = call "Q Driver.vi"("error in (no error)"=w509, "Q Operation"=Queue_Operation_Mode."Flush Q") -> ("error out"=w507:errorcluster)  [unwired: 12 in, 1 out]
            n208 = call "Q Driver.vi"("State In"="Exit" ("States[]"), "error in (no error)"=w507, "Q Operation"=Queue_Operation_Mode."Enqueue") -> ("error out"=w506:errorcluster)  [unwired: 11 in, 1 out]
          }
          frame True {
            # "Continue"
          }
        }
      }
      frame "/***----------Exit----------***/" {
      }
      frame "Exit" {
        # "Exit the State Machine"
        n209 = call "Q Driver.vi"("error in (no error)"=w518, "Q Operation"=Queue_Operation_Mode."Flush Q") -> ("error out"=w517:errorcluster)  [unwired: 12 in, 1 out]
        n210 = call "Q Driver.vi"("error in (no error)"=w517, "Q Operation"=Queue_Operation_Mode."Close Q") -> ("error out"=w516:errorcluster)  [unwired: 12 in, 1 out]
      }
    }
  }
  "error out" <- w8
